vi "SQL Builder.vi"(8 "error in":errorcluster, 11 "SELECTED COLUMNS":string[](array[string])) -> (3 "Built Query":string)   [LabVIEW 2020]
uses:
  <vilib>/regexp/Match Regular Expression.xnode
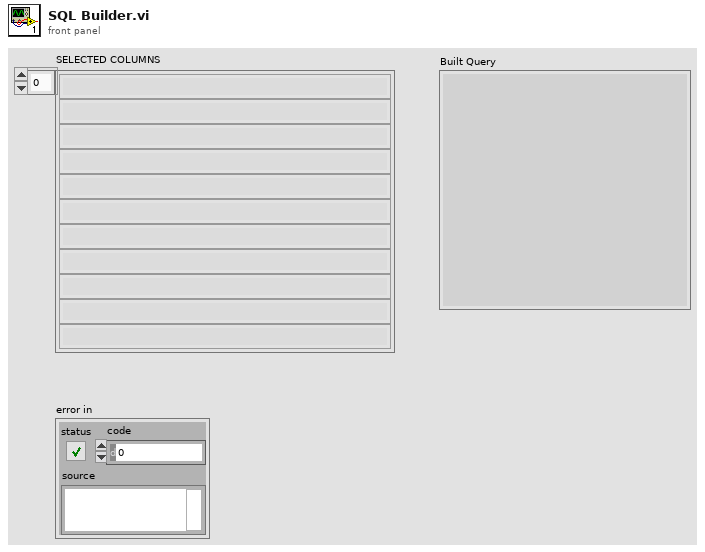
[diagram p1: front panel]
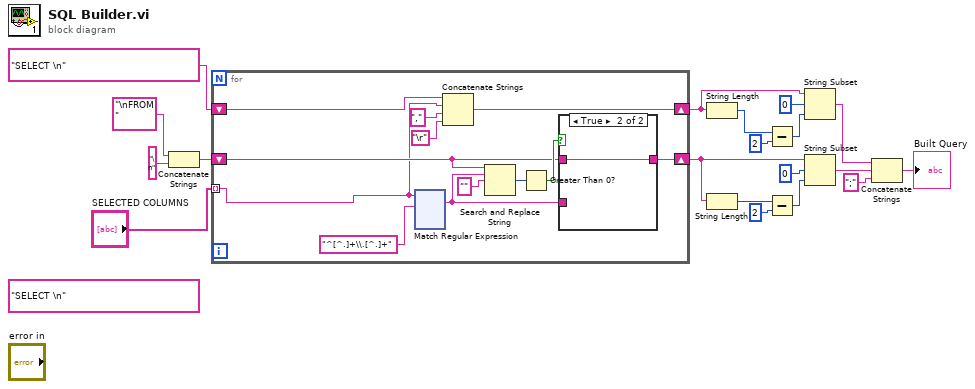
[diagram p0: block diagram]
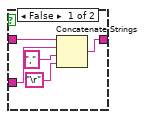
[diagram p2: hidden frame]
diagram:
  (unwired) "SELECT \n"
  n1 = Concatenate Strings("\nFROM " ("string"), "\n" ("string")) -> (w12:string)
  n2 = for {
    tunnel: "SELECTED COLUMNS" -> [w20] mode=indexing
    shift-right: [w29] -> w15
    shift-left: "SELECT \n" -> [w28]
    shift-right: [w21] -> w10
    shift-left: w12 -> [w22]
    n3 = xnode "Match Regular Expression"("input string"=w20, "regular expression"="^[^.]+\\.[^.]+") -> ("whole match"=w26:string)  [unwired: 4 in, 4 out]
    n4 = Concatenate Strings(w28, w20, "," ("string"), "\r") -> (w29:string)
    n5 = Search and Replace String(input string=w22, search string=w26, replace string="" ("replace string (\"\")")) -> (number of replacements=w24:i32)  [unwired: 5 in, 3 out]
    n6 = Greater Than 0?(x=w24) -> (x > 0?=w23:bool)
    n7 = case shown="True" w23 {
      tunnel: w26 -> [w33 _]
      tunnel: w22 -> [w34 w37]
      tunnel: [w32 w37] -> w21
      frame False {
        n8 = Concatenate Strings(w34, w33, "," ("string"), "\r") -> (w32:string)
      }
      frame True {
      }
    }
  }
  n9 = String Length(string=w15) -> (length=w6:i32)
  n10 = String Length(string=w10) -> (length=w2:i32)
  n11 = Subtract(x=w6, y=2) -> (x-y=w4:i32)
  n12 = Subtract(x=w2, y=2) -> (x-y=w1:i32)
  n13 = String Subset(string=w15, offset (0)=0, length (rest)=w4) -> (substring=w17:string)
  n14 = String Subset(string=w10, offset (0)=0, length (rest)=w1) -> (substring=w9:string)
  n15 = Concatenate Strings(w17, w9, ";" ("string")) -> (→"Built Query":string)
